vi "TimedReadFromTextFileVI.vi"(7 "Sample Rate (kHz)":i64=25, 13 "dt":dbl=4e-05, 14 "stop in":bool) -> (4 "Search Pattern":string, 6 "offset (in bytes) 2":i64, 8 "Waveform":waveform(dbl), 15 "error out":errorcluster)   [LabVIEW 2022 SP3]
uses:
  <vilib>/Platform/TimedLoop/XDataNode/timing_clust.ctl
  <vilib>/Platform/TimedLoop/XDataNode/nitl_modes.ctl
  <vilib>/Platform/TimedLoop/XDataNode/wakeup.ctl
  <vilib>/Platform/TimedLoop/scheduler/LVUserAPI/_suppVIs/Create_1kHz_TSource.vi
  <vilib>/platform/TimedLoop/XDataNode/XDataNode.xnode
  <vilib>/Platform/TimedLoop/XDataNode/XDNodeRunTimeDep.lvlib
panel:
  in  "Cluster 3":T1={"Path txt/csv File"=path "C:/Users/LAV-UFSC/Documents/LAV - TCC/acc_time/Previous Data/handlebar_acc1_run1.txt", "Delimiter"=".", "Separator"="\\t", "Offset (lines)"=21.0, "string"="3e", "format string"="%^", "access (0:read/write)"=enum."read/write", "operation (0:open)"=enum."open"}
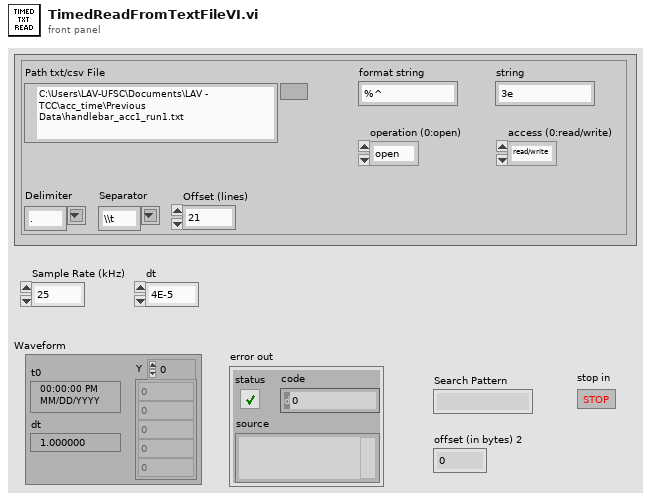
[diagram p1: front panel]
types:
  T1 = cluster{"Path txt/csv File":path, "Delimiter":string, "Separator":string, "Offset (lines)":dbl, "string":string, "format string":string, "access (0:read/write)":enum16{"read/write", "read-only", "write-only"}, "operation (0:open)":enum16{"open", "replace", "create", "open or create", "replace or create", "replace or create with confirmation"}}
  T2 = enum16{"open", "replace", "create", "open or create", "replace or create", "replace or create with confirmation"}
  T3 = typedef "XDNodeRunTimeDep.lvlib/timing_clust.ctl" = cluster{"Expected End [f-1]":u64, "Actual End [f-1]":u64, "Finished Late? [f-1]":bool, "Expected End [i-1]":u64, "Actual End [i-1]":u64, "Finished Late? [i-1]":bool, "Expected Start [i]":u64, "Actual Start [i]":u64, "Expected Start [f]":u64, "Actual Start [f]":u64, "Source Name":string, "Structure Name":string, "Period":i64, "Deadline":i64, "Offset":i64, "Start":i64, "Priority":i32, "Timeout":i32, "Mode":T4, "Wakeup Reason":T5, "Error":errorcluster, "Source Type":string, "Secondary Source Type":string, "Global End Time":u64, "Global Start Time":u64, "Frame Duration":u64, "Iteration Duration":u64, "Assigned CPU":i32, "I/O Scan Engine Mode":u32}
  T4 = typedef "XDNodeRunTimeDep.lvlib/nitl_modes.ctl" = enum32{"No Change", "Process missed periods, maintain original phase", "Discard missed periods, maintain original phase", "Process missed periods, ignore original phase", "Discard missed periods, ignore original phase"}
  T5 = typedef "XDNodeRunTimeDep.lvlib/wakeup.ctl" = enum32{"Normal", "Aborted", "Asynchronous wakeup", "Timing source error", "Timed loop error", "Timeout"}
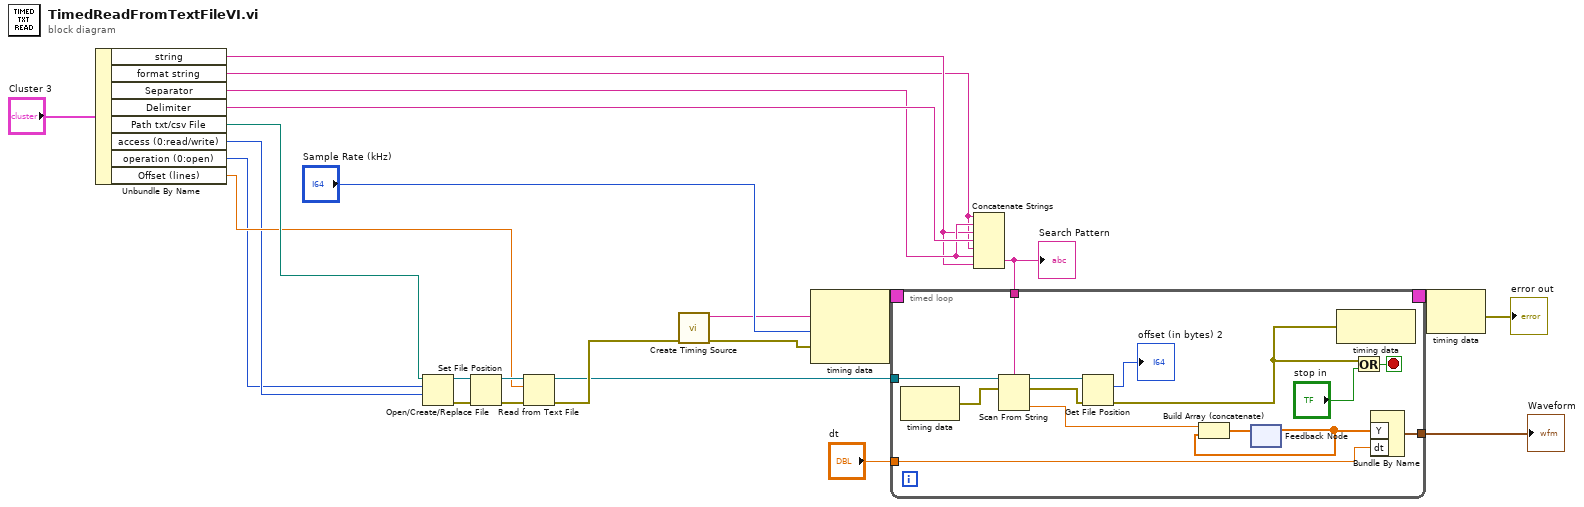
[diagram p0: block diagram]
diagram:
  n1 = Unbundle By Name("Cluster 3") -> ("string"=w5:string, "format string"=w4:string, "Separator"=w6:string, "Delimiter"=w8:string, "Path txt/csv File"=w7:path, "access (0:read/write)"=w2:enum16{"read/write", "read-only", "write-only"}, "operation (0:open)"=w1:T2, "Offset (lines)"=w3:dbl)
  n2 = Open/Create/Replace File(file path (use dialog)=w7, operation (0:open)=w1, access (0:read/write)=w2) -> (refnum out=w14:refnum<file>, error out=w12:errorcluster)  [unwired: 3 in, 1 out]
  n3 = Set File Position(refnum=w14, error in=w12) -> (refnum out=w13:refnum<file>, error out=w19:errorcluster)  [unwired: 2 in]
  n4 = Read from Text File(file (use dialog)=w13, count=w3, error in=w19) -> (refnum out=w20:refnum<file>, error out=w21:errorcluster)  [unwired: 1 in, 2 out]
  n5 = call-poly <vilib>:"Create Timing Source.vi"("error in (no error)"=w21) -> ("error out"=w16:errorcluster, "name (out)"=w15:string)  [unwired: 9 in]
  n6 = node-c288(w15, "Sample Rate (kHz)", w16) -> (w24:T3)
  n7 = Concatenate Strings(w4, w6, w5, w8, w4, w6, w5) -> (w18:string)
  "Search Pattern" <- w18
  n8 = timed-loop {
    timing: w24 -> [_]
    timing-out: [_] -> w23
    tunnel: w18 -> [w32]
    tunnel: w20 -> [w31]
    tunnel: "dt" -> [w27]
    tunnel: [w26] -> w10
    stop <- w33 stop-if-true
    n9 = node-c288() -> (w30:errorcluster)  [unwired: 1 in]
    n10 = Scan From String(w32, w31, w30) -> (w38:refnum<file>, w37:errorcluster, output 2=w35:dbl)  [unwired: 3 in]
    n11 = Get File Position(4:w37, 7:w38) -> (0:w29:errorcluster, 2:→"offset (in bytes) 2":i64)  [unwired: 1 out]
    n12 = feedback #1() -> (w25:dbl[])  [unwired: 1 in]
    n13 = Build Array (concatenate)(w35, w25) -> (w34:dbl[])
    n14 = feedback-in #1(w34) -> ()
    n15 = node-c288(w29) -> ()  [unwired: 1 out]
    n16 = Or(x=w29, y="stop in") -> (x .or. y?=w33:bool)
    n17 = Bundle By Name("Y"=w25, "dt"=w27) -> (w26:waveform(dbl))  [unwired: 1 in]
  }
  "Waveform" <- w10
  n18 = node-c288(w23) -> (→"error out":errorcluster)
